vi "OPC test (original from forum).vi"() -> ()   [LabVIEW 2024]
uses:
  <vilib>/Utility/Data Type/Type Definitions/Data Type.ctl
  System.Xml
  C:/Users/ban106/Downloads/NuGetPackages/OpcNetApi.dll
  ban106/Downloads/NuGetPackages/OpcNetApi.dll
  <vilib>/Utility/Data Type/NI_Data Type.lvlib
  C:/Users/ban106/Downloads/NuGetPackages/OpcNetApi.Com.dll
  ban106/Downloads/NuGetPackages/OpcNetApi.Com.dll
panel:
  out "Read ResultID":string
  out "ResultID":string[](array[string])
  out "server status":T1
  out "server properties":T2
  out "type":T3
  out "kHz":dbl
  in  "stop":bool
  out "variant":variant
  out "ItemName":string
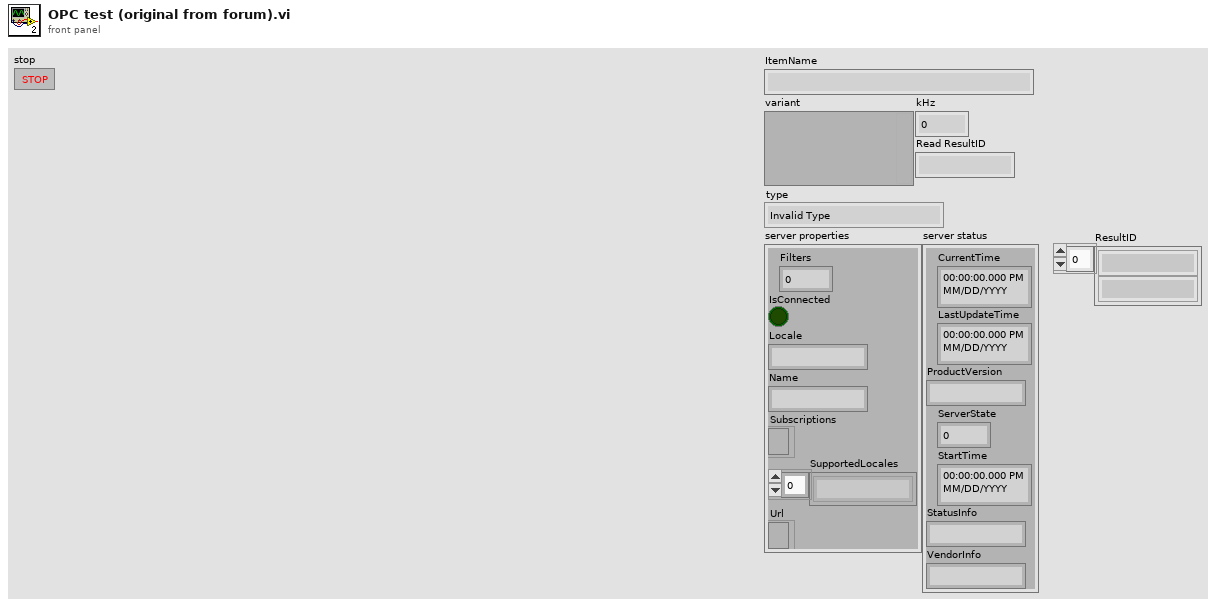
[diagram p1: front panel]
types:
  T1 = cluster{"CurrentTime":timestamp, "LastUpdateTime":timestamp, "ProductVersion":string, "ServerState":i32, "StartTime":timestamp, "StatusInfo":string, "VendorInfo":string}
  T2 = cluster{"Filters":i32, "IsConnected":bool, "Locale":string, "Name":string, "Subscriptions":refnum<k24>, "SupportedLocales":string[], "Url":refnum<k24>}
  T3 = typedef "NI_Data Type.lvlib/Data Type.ctl" = enum8{"Invalid Type", "Void", "I8", "I16", "I32", "I64", "U8", "U16", "U32", "U64", "Single Float", "Double Float", "Extended Float", "Single Complex", "Double Complex", "Extended Complex", "Enum U8", "Enum U16", "Enum U32", "Enum U64", "Single Float With Unit", "Double Float With Unit", "Extended Float With Unit", "Single Complex with Unit", "Double Complex with Unit", "Extended Complex with Unit", "Boolean", "String", "Path", "Picture", "Tag", "Array", "Cluster", "Variant", "LV Variant", "Waveform", "Timestamp", "Digital Waveform", "Digital Data", "ExpressData", "Refnum", "External Data", "VI", "Poly VI", "LabVIEW Class Instance", "Fixed Point", "Set Collection", "Map Collection"}
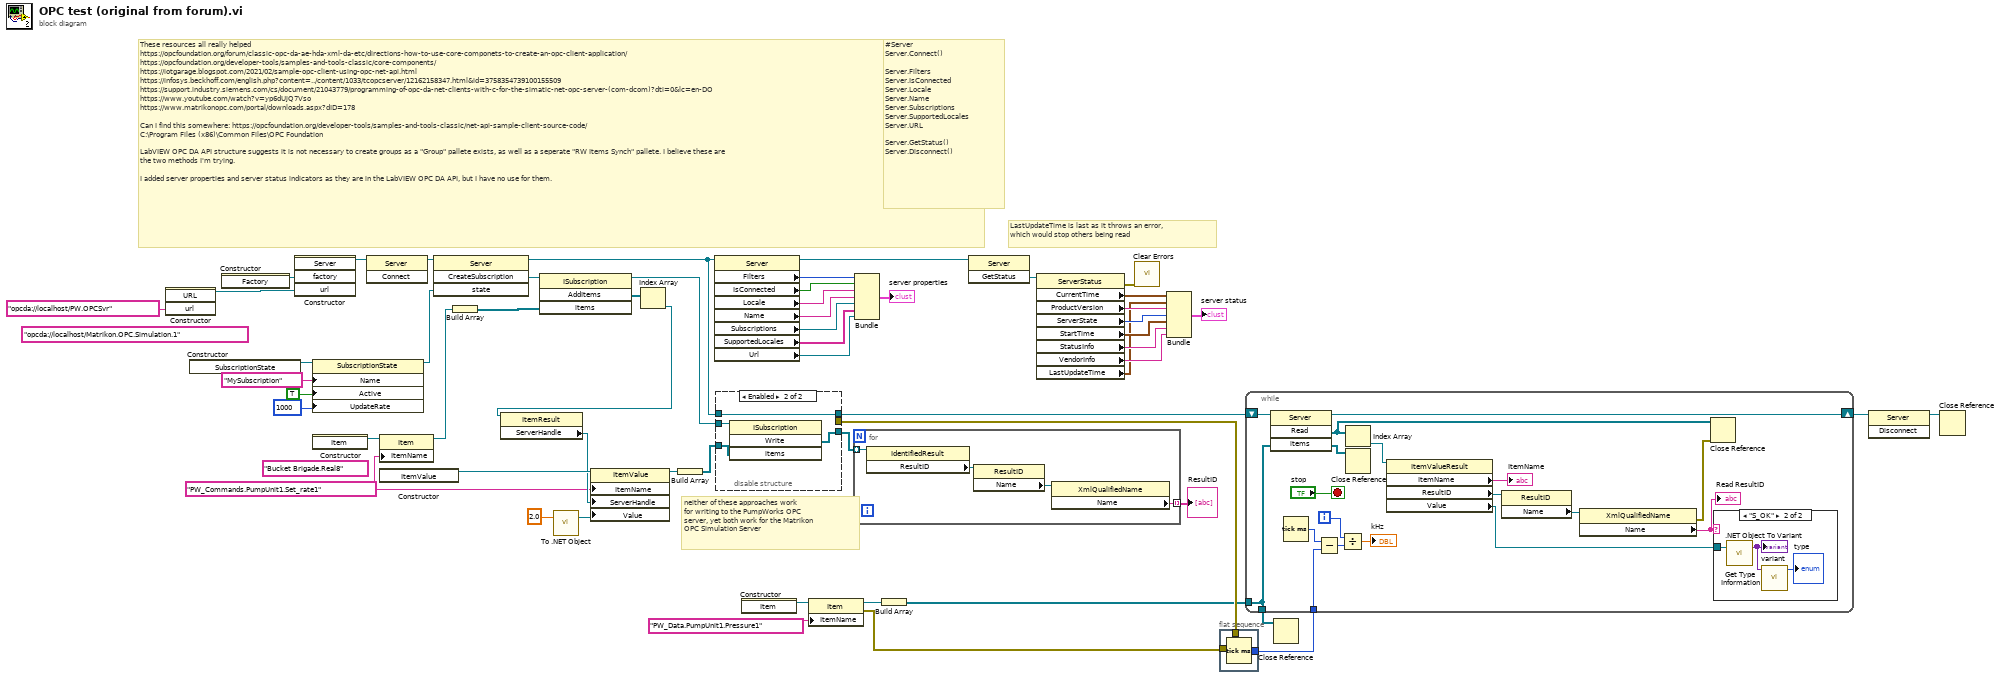
[diagram p0: block diagram]
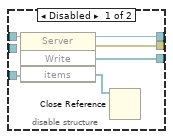
[diagram p2: hidden frame]
diagram:
  (unwired) "Bucket Brigade.Real8" ("itemName")
  (unwired) "opcda://localhost/Matrikon.OPC.Simulation.1" ("url")
  w3 = "PW_Commands.PumpUnit1.Set_rate1" ("itemName")
  # "neither of these approaches work\nfor writing to the PumpWorks OPC\nserver, yet both work for the Matrikon\nOPC Simulation Server"
  # "LastUpdateTime is last as it throws an error,\nwhich would stop others being read"
  # "#Server\nServer.Connect()\n\nServer.Filters\nServer.IsConnected\nServer.Locale\nServer.Name\nServer.Subscriptions\nServer.SupportedLocales\nServer.URL\n\nServer.GetStatus()\nServer.Disconnect()"
  # "These resources all really helped\nhttps://opcfoundation.org/forum/classic-opc-da-ae-hda-xml-da-etc/directions-how-to-use-core-componets-to-create-an-opc-client-application/\nhttps://opcfoundation.org/developer-tools/samples-and-tools-classic/core-components/\nhttps://iotgarage.blogspot.com/2021/02/sample-opc-client-using-opc-net-api.html\nhttps://infosys.beckhoff.com/english.php?content=../content/1033/tcopcserver/12162158347.html&id=3758354739100155509\nhttps://support.industry.siemens.com/cs/document/21043779/programming-of-opc-da-net-clients-with-c-for-the-simatic-net-opc-server-(com-dcom)?dti=0&lc=en-DO\nhttps://www.youtube.com/watch?v=yp6dUjQ7Vso\nhttps://www.matrikonopc.com/portal/downloads.aspx?dID=178\n\nCan I find this somewhere: https://opcfoundation.org/developer-tools/samples-and-tools-classic/net-api-sample-client-source-code/\nC:\\Program Files (x86)\\Common Files\\OPC Foundation\n\nLabVIEW OPC DA API structure suggests it is not necessary to create groups as a \"Group\" pallete exists, as well as a seperate \"RW Items Synch\" pallete. I believe these are\nthe two methods I'm trying.\n\nI added server properties and server status indicators as they are in the LabVIEW OPC DA API, but I have no use for them."
  n1 = constructor class="URL"("url"="opcda://localhost/PW.OPCSvr") -> (reference out=w57:refnum<k24>)  [unwired: 3 in, 3 out]
  n2 = constructor class="SubscriptionState"() -> (reference out=w39:refnum<k24>)  [unwired: 3 in, 2 out]
  n3 = constructor class="Factory"() -> (reference out=w56:refnum<k24>)  [unwired: 3 in, 2 out]
  n4 = constructor class="Server"("factory"=w56, "url"=w57) -> (reference out=w55:refnum<k24>)  [unwired: 3 in, 4 out]
  n5 = property class="SubscriptionState"(reference=w39, "Name"="MySubscription", "Active"=TRUE, "UpdateRate"=1000) -> (reference out=w34:refnum<k24>)  [unwired: 1 in, 1 out]
  n6 = constructor class="Item"() -> (reference out=w36:refnum<k24>)  [unwired: 3 in, 2 out]
  n7 = invoke class="Server" method="Connect"(reference=w55) -> (reference out=w35:refnum<k24>)  [unwired: 2 in, 2 out]
  n8 = property class="Item"(reference=w36, "ItemName"=w3) -> (reference out=w32:refnum<k24>)  [unwired: 1 in, 1 out]
  n9 = constructor class="ItemValue"() -> (reference out=w50:refnum<k24>)  [unwired: 3 in, 2 out]
  n10 = invoke class="Server" method="CreateSubscription"(reference=w35, "state"=w34) -> (reference out=w29:refnum<k24>, "CreateSubscription"=w33:refnum<k24>)  [unwired: 2 in, 2 out]
  n11 = Build Array(w32) -> (w31:refnum<k24>[])
  n12 = invoke class="ISubscription" method="AddItems"(reference=w33, "items"=w31) -> (reference out=w30:refnum<k24>, "AddItems"=w6:refnum<k24>[])  [unwired: 2 in, 2 out]
  n13 = call <vilib>:"To .NET Object.vi"("anything"=sgl 2.0) -> (".NET object"=w46:refnum<k24>)  [unwired: 1 in, 1 out]
  n14 = Index Array(array=w6) -> (element=w5:refnum<k24>)  [unwired: 1 in]
  n15 = property class="ItemResult"(reference=w5) -> ("ServerHandle"=w4:refnum<k24>)  [unwired: 1 in, 2 out]
  n16 = property class="ItemValue"(reference=w50, "ItemName"=w3, "ServerHandle"=w4, "Value"=w46) -> (reference out=w49:refnum<k24>)  [unwired: 1 in, 1 out]
  n17 = Build Array(w49) -> (w47:refnum<k24>[])
  n18 = property class="Server"(reference=w29) -> (reference out=w20:refnum<k24>, "Filters"=w28:i32, "IsConnected"=w27:bool, "Locale"=w26:string, "Name"=w25:string, "Subscriptions"=w24:refnum<k24>, "SupportedLocales"=w23:string[], "Url"=w22:refnum<k24>)  [unwired: 1 in, 1 out]
  n19 = disable-structure shown="Enabled" {
    disable-tunnel: [w63 _] -> w51
    disable-tunnel: [w62 w65] -> w48
    disable-tunnel: w47 -> [w61 w67]
    disable-tunnel: w29 -> [w59 w65]
    disable-tunnel: w30 -> [_ w66]
    disable-tunnel: [w58 w64] -> w8
    frame Disabled {
      n20 = invoke class="Server" method="Write"(reference=w59, "items"=w61) -> (reference out=w62:refnum<k24>, error out=w63:errorcluster, "Write"=w58:refnum<k24>[], "items"=w60:refnum<k24>[])  [unwired: 2 in]
      n21 = Close Reference(reference=w60) -> ()  [unwired: 1 in, 1 out]
    }
    frame Enabled {
      n22 = invoke class="ISubscription" method="Write"(reference=w66, "items"=w67) -> ("Write"=w64:refnum<k24>[])  [unwired: 2 in, 3 out]
    }
  }
  n23 = constructor class="Item"() -> (reference out=w44:refnum<k24>)  [unwired: 3 in, 2 out]
  n24 = property class="Item"(reference=w44, "ItemName"="PW_Data.PumpUnit1.Pressure1" ("itemName")) -> (reference out=w43:refnum<k24>, error out=w42:errorcluster)  [unwired: 1 in]
  n25 = for {
    tunnel: w8 -> [w71] mode=indexing
    tunnel: [w68] -> w7 mode=indexing
    n26 = property class="IdentifiedResult"(reference=w71) -> ("ResultID"=w70:refnum<k24>)  [unwired: 1 in, 2 out]
    n27 = property class="ResultID"(reference=w70) -> ("Name"=w69:refnum<k24>)  [unwired: 1 in, 2 out]
    n28 = property class="XmlQualifiedName"(reference=w69) -> ("Name"=w68:string)  [unwired: 1 in, 2 out]
  }
  "ResultID" <- w7
  n29 = Bundle("Filters"=w28, "IsConnected"=w27, "Locale"=w26, "Name"=w25, "Subscriptions"=w24, "SupportedLocales"=w23, "Url"=w22) -> (→"server properties":T2)  [unwired: 1 in]
  n30 = Build Array(w43) -> (w41:refnum<k24>[])
  n31 = invoke class="Server" method="GetStatus"(reference=w20) -> ("GetStatus"=w19:refnum<k24>)  [unwired: 2 in, 2 out]
  n32 = property class="ServerStatus"(reference=w19) -> (error out=w10:errorcluster, "CurrentTime"=w18:timestamp, "ProductVersion"=w17:string, "ServerState"=w16:i32, "StartTime"=w15:timestamp, "StatusInfo"=w14:string, "VendorInfo"=w13:string, "LastUpdateTime"=w12:timestamp)  [unwired: 1 in, 1 out]
  n33 = call <vilib>:"Clear Errors.vi"("error in (no error)"=w10) -> ()  [unwired: 5 in, 2 out]
  n34 = Bundle("CurrentTime"=w18, "LastUpdateTime"=w12, "ProductVersion"=w17, "ServerState"=w16, "StartTime"=w15, "StatusInfo"=w14, "VendorInfo"=w13) -> (→"server status":T1)  [unwired: 1 in]
  n35 = flat-sequence {
    tunnel: w51 -> [_]
    tunnel: w42 -> [_]
    tunnel: [w72] -> w53
    frame #0 {
      n36 = Tick Count (ms)() -> (millisecond timer value=w72:u32)
    }
  }
  n37 = while {
    shift-right: [w88] -> w54
    shift-left: w48 -> [w90]
    tunnel: w53 -> [w83]
    tunnel: w41 -> [w77]
    tunnel: [w77] -> w40
    i -> [w81]
    stop <- "stop" stop-if-true
    n38 = invoke class="Server" method="Read"(reference=w90, "items"=w77) -> (reference out=w88:refnum<k24>, "Read"=w78:refnum<k24>[], "items"=w79:refnum<k24>[])  [unwired: 2 in, 1 out]
    n39 = Tick Count (ms)() -> (millisecond timer value=w84:u32)
    n40 = Subtract(x=w84, y=w83) -> (x-y=w82:u32)
    n41 = Divide(x=w81, y=w82) -> (x/y=→"kHz":dbl)
    n42 = Index Array(array=w78) -> (element=w89:refnum<k24>)  [unwired: 1 in]
    n43 = Close Reference(reference=w79) -> ()  [unwired: 1 in, 1 out]
    n44 = property class="ItemValueResult"(reference=w89) -> ("ItemName"=→"ItemName":string, "ResultID"=w75:refnum<k24>, "Value"=w86:refnum<k24>)  [unwired: 1 in, 2 out]
    n45 = property class="ResultID"(reference=w75) -> ("Name"=w76:refnum<k24>)  [unwired: 1 in, 2 out]
    n46 = property class="XmlQualifiedName"(reference=w76) -> (error out=w73:errorcluster, "Name"=w74:string)  [unwired: 1 in, 1 out]
    "Read ResultID" <- w74
    n47 = Close Reference(reference=w78, error in (no error)=w73) -> ()  [unwired: 1 out]
    n48 = case shown="\"S_OK\"" w74 {
      tunnel: w86 -> [_ w93]
      frame Default {
      }
      frame "S_OK" {
        n49 = call <vilib>:".NET Object To Variant.vi"(".NET object"=w93) -> ("variant"=w92:variant)  [unwired: 1 in, 1 out]
        "variant" <- w92
        n50 = call <vilib>:"Get Type Information.vi"("variant"=w92) -> ("type"=→"type":T3)  [unwired: 6 in, 4 out]
      }
    }
  }
  n51 = Close Reference(reference=w40) -> ()  [unwired: 1 in, 1 out]
  n52 = invoke class="Server" method="Disconnect"(reference=w54) -> (reference out=w52:refnum<k24>)  [unwired: 2 in, 2 out]
  n53 = Close Reference(reference=w52) -> ()  [unwired: 1 in, 1 out]
